vi "Reset_Timer.vi"(8 "error in (no error)":errorcluster, 11 "Timer_Event in":refnum<class "Timer_Event.lvclass">) -> (0 "error out":errorcluster, 3 "Timer_Event out":refnum<class "Timer_Event.lvclass">)   [LabVIEW 2020, in "Timer_Event.lvlib" / "Timer_Event.lvclass"]
uses:
  Timer_Event.lvclass
  Timer_Event.lvclass/Timer_Event.ctl
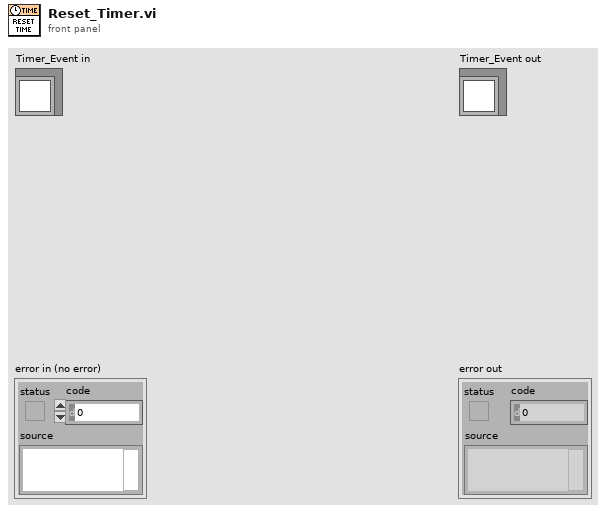
[diagram p1: front panel]
types:
  T1 = cluster{"Start Time":u32, "Elapsed Time":u32, "Running":bool}
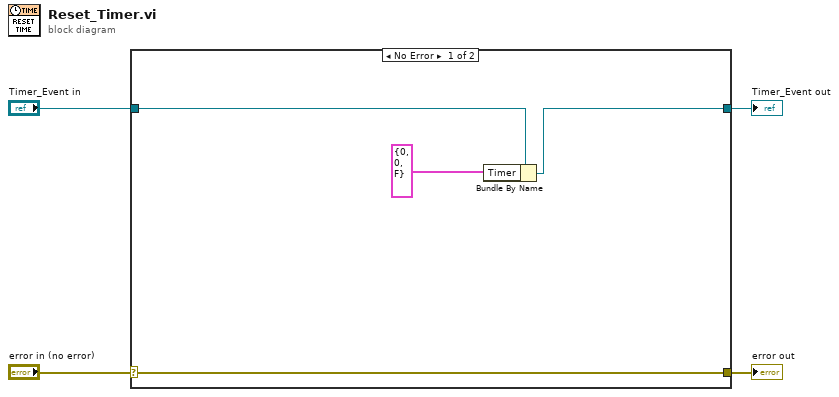
[diagram p0: block diagram]
diagram:
  n1 = case shown="No Error" "error in (no error)" {
    selector: "error in (no error)" -> [w8 w10]
    tunnel: [w8 w10] -> w3
    tunnel: [w5 w9] -> w1
    tunnel: "Timer_Event in" -> [w7 w9]
    frame No Error {
      n2 = Bundle By Name(cluster=w7, "Timer"=T1 {"Start Time"=0, "Elapsed Time"=0, "Running"=FALSE}) -> (w5:refnum<class "Timer_Event.lvclass">)
    }
    frame Error {
    }
  }
  "error out" <- w3
  "Timer_Event out" <- w1
